vi "Receive Message.vi"(6 "priority":i32, 10 "IModel in":refnum<class "IModel.lvclass">, 11 "Message in":refnum<class "Message.lvclass">) -> (0 "error out":errorcluster, 2 "Actor out":refnum<class "Actor.lvclass">)   [LabVIEW 2019, in "IModel.lvlib" / "IModel.lvclass"]
uses:
  <vilib>/gpm_packages/@cs/mva-core/Source/IModel/IModel/IModel.lvclass
  <vilib>/ActorFramework/Message/Message.lvclass
  <vilib>/ActorFramework/Actor/Actor.lvclass
  C:/Program Files/National Instruments/LabVIEW 2019/vi.lib/ActorFramework/Actor/Actor.lvclass
  C:/Program Files/National Instruments/LabVIEW 2019/vi.lib/gpm_packages/@cs/mva-core/Source/IObserver/IObserver/IObserver.lvclass
  <vilib>/ActorFramework/Stop Msg/Stop Msg.lvclass
  C:/Program Files/National Instruments/LabVIEW 2019/vi.lib/ActorFramework/Message/Message.lvclass
  <vilib>/gpm_packages/@cs/mva-core/Source/IModel/IModel/IModel.lvclass/IModel.ctl
  <vilib>/ActorFramework/Message Enqueuer/Message Enqueuer.lvclass/Message Enqueuer.ctl
  <vilib>/gpm_packages/@cs/mva-core/Source/IObserver/IObserver/IObserver.lvclass/IObserver.ctl
  <vilib>/gpm_packages/@cs/event-logger/Source/Composed Log/LoggerReference/LoggerReference.lvclass/LoggerReference.ctl
  <vilib>/ActorFramework/Stop Msg/Send Normal Stop.vi
  <vilib>/gpm_packages/@cs/mva-core/Source/IObserver/IObserver/Log Framework Event.vi
  <vilib>/ActorFramework/Message Enqueuer/Enqueue.vi
  <vilib>/gpm_packages/@cs/event-logger/Source/Composed Log/LoggerReference/Log Event.vi
  <vilib>/gpm_packages/@cs/event-logger/Source/Composed Log/LoggerReference/Log.vi
  <vilib>/gpm_packages/@cs/event-logger/Source/Composed Log/LoggerReference/Get Valid Event Time.vi
  <vilib>/gpm_packages/@cs/event-logger/Source/Composed Log/LoggerReference/Remove Stale Logs.vi
  <vilib>/ActorFramework/Message Priority Queue/Priority Enqueue.vi
  <vilib>/Utility/LVClass/Get LV Class Name.vi
  <vilib>/ActorFramework/Message Enqueuer/Message Enqueuer.lvclass
  <vilib>/gpm_packages/@cs/mva-core/Source/IObserver/IObserver/IObserver.lvclass
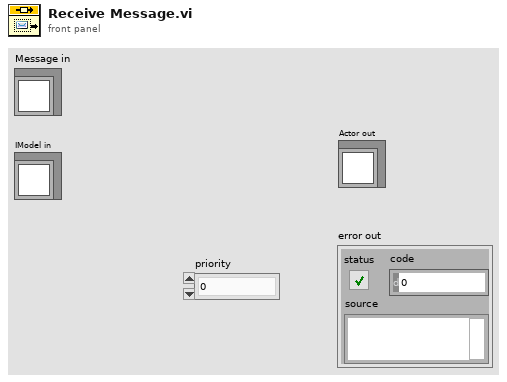
[diagram p1: front panel]
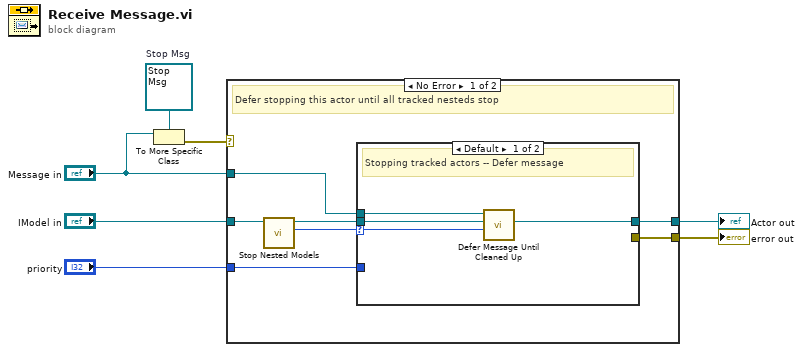
[diagram p0: block diagram]
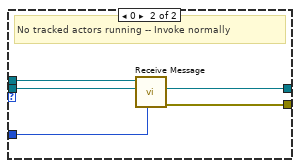
[diagram p2: hidden frame]
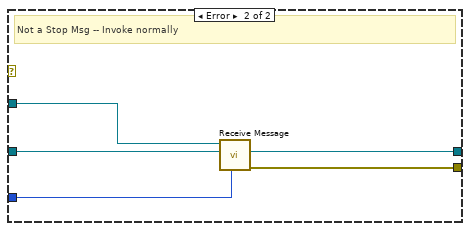
[diagram p3: hidden frame]
diagram:
  w3 = refnum<class "Stop Msg.lvclass"> refnum  # Stop Msg
  n1 = To More Specific Class(target class=w3, reference="Message in") -> (error out=w2:errorcluster)  [unwired: 1 in, 1 out]
  n2 = case shown="No Error" w2 {
    tunnel: [w14 w28] -> w7
    tunnel: [w12 w27] -> w6
    tunnel: "priority" -> [w10 w26]
    tunnel: "IModel in" -> [w13 w25]
    tunnel: "Message in" -> [w11 w24]
    frame No Error {
      # "Defer stopping this actor until all tracked nesteds stop"
      n3 = call <vilib>:"Stop Nested Models.vi"("IModel in"=w13) -> ("Tracked Actors Running"=w8:i32, "IModel out"=w9:refnum<class "IModel.lvclass">)  [unwired: 8 in, 1 out]
      n4 = case shown="Default" w8 {
        selector: w8 -> [w15 _]
        tunnel: [_ w21] -> w14
        tunnel: [w18 w22] -> w12
        tunnel: w11 -> [w17 w23]
        tunnel: w10 -> [_ w20]
        tunnel: w9 -> [w16 w19]
        frame Default {
          # "Stopping tracked actors -- Defer message"
          n5 = call <vilib>:"Defer Message Until Cleaned Up.vi"("Tracked Actor Count"=w15, "IModel in"=w16, "Message in"=w17) -> ("IModel out"=w18:refnum<class "IModel.lvclass">)  [unwired: 8 in]
        }
        frame 0 {
          # "No tracked actors running -- Invoke normally"
          n6 = call-parent "Receive Message.vi"("priority"=w20, "Actor in"=w19, "Message in"=w23) -> ("error out"=w21:errorcluster, "Actor out"=w22:refnum<class "Actor.lvclass">)  [unwired: 7 in]
        }
      }
    }
    frame Error {
      # "Not a Stop Msg -- Invoke normally"
      n7 = call-parent "Receive Message.vi"("priority"=w26, "Actor in"=w25, "Message in"=w24) -> ("error out"=w28:errorcluster, "Actor out"=w27:refnum<class "Actor.lvclass">)  [unwired: 7 in]
    }
  }
  "error out" <- w7
  "Actor out" <- w6
